vi "Hault.vi"(7 "Device Number":T1) -> ()   [LabVIEW 2016, in "navX Library.lvlib"]
uses:
  _TypeDefs/FRIC_navX_DeviceNumbersTypeDef.ctl
  _TypeDefs/Z900_navX_ActionTypeDef.ctl
  navX Library.lvlib
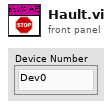
[diagram p1: front panel]
types:
  T1 = typedef "navX Library.lvlib/FRIC_navX_DeviceNumbersTypeDef.ctl" = enum16{"Dev0", "Dev1", "Dev2", "Dev3"}
  T2 = typedef "navX Library.lvlib/Z900_navX_ActionTypeDef.ctl" = enum16{"None", "Halt", "Normal Read", "Update Serial Protocol", "Update Rate Htz", "Zero-Yaw", "Zero-Displacement", "Zero-Velocity"}
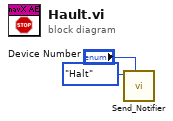
[diagram p0: block diagram]
diagram:
  n1 = call "Send_Notifier.vi"("Device Number"="Device Number", "navX Action"=Z900_navX_ActionTypeDef."Halt") -> ()  [unwired: 10 in]
